vi "RB2 find red 3 dot.vi"(0 "Image In":T1, 1 "error in":errorcluster) -> (2 "Image Out":T1, 3 "Num of\nRed Dots":i32, 4 "Red Dot\nLocation":T2(array[cluster]), 5 "error out":errorcluster)   [LabVIEW 2012]
doc: "This VI find a RED dot on the vehicle in the Mars landscape for Robotics II Spring 2014. It reports the number of Red dots found and their location."
uses:
  <vilib>/vision/Image Controls.llb/IMAQ Image.ctl
  <vilib>/vision/NI_Vision_Development_Module.lvlib
panel:
  out "Mars Result":T1(plugin-control)
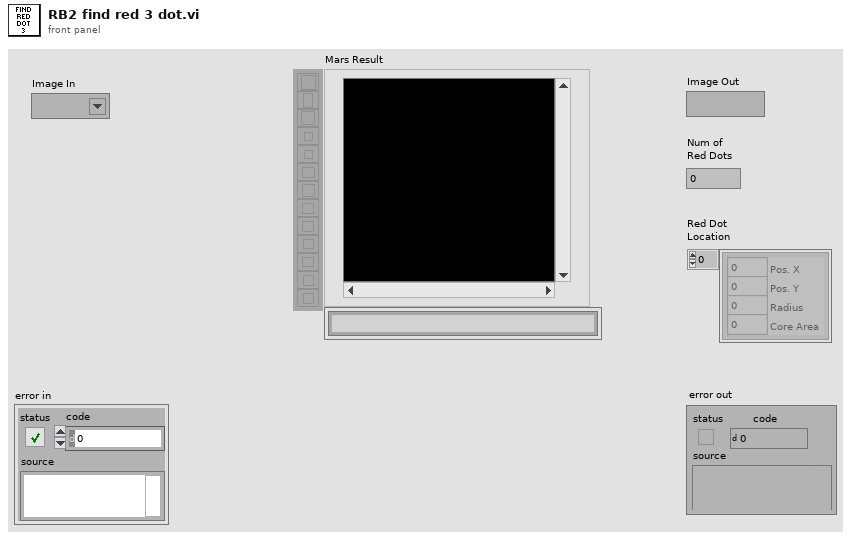
[diagram p1: front panel]
types:
  T1 = typedef "IMAQ Image.ctl" = refnum<image>
  T2 = cluster{"Pos. X":i32, "Pos. Y":i32, "Radius":i32, "Core Area":i32}[]
  T3 = enum32{"AutoM", "Close", "Dilate", "Erode", "Gradient", "Gradient in", "Gradient out", "HitMiss", "Open", "PClose", "POpen", "Thick", "Thin"}
  T4 = typedef "Image Type" = u32
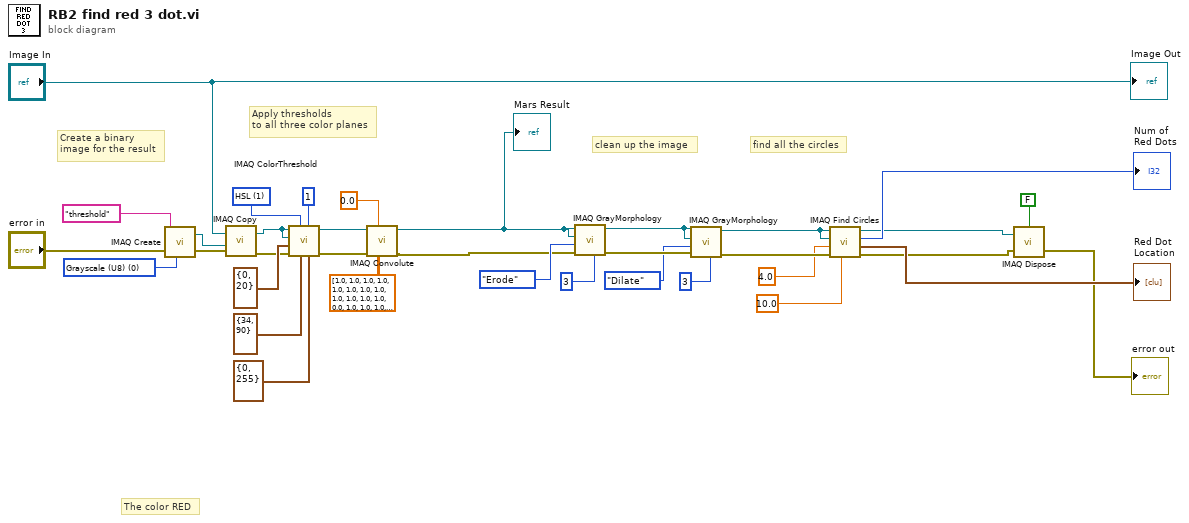
[diagram p0: block diagram]
diagram:
  w12 = u16 1 items=["RGB", "HSL", "HSV", "HSI"] ("Color Mode")
  w32 = T4 0 items=["Grayscale (U8)", "Grayscale (I16)", "Grayscale (SGL)", "Complex (CSG)", "RGB (U32)", "HSL (U32)", "RGB (U64)", "Grayscale (U16)"] ("Image Type")
  # "Create a binary\nimage for the result"
  # "The color RED"
  # "Apply thresholds\nto all three color planes"
  # "find all the circles"
  # "clean up the image"
  n1 = call "IMAQ Create"("Image Name"="threshold", "Image Type"=w32, "error in (no error)"="error in") -> ("New Image"=w34:T1, "error out"=w33:errorcluster)  [unwired: 2 in]
  n2 = call "IMAQ Copy"("error in (no error)"=w33, "Image Dst"=w34, "Image Src"="Image In") -> ("error out"=w3:errorcluster, "Image Dst Out"=w4:T1)  [unwired: 3 in]
  n3 = call "IMAQ ColorThreshold"("Blue or Luma or Val or Inten Range"=cluster{"Lower value":i32, "Upper value":i32} {"Lower value"=0, "Upper value"=255}, "Replace Value"=1, "Green or Sat Range"=cluster{"Lower value":i32, "Upper value":i32} {"Lower value"=34, "Upper value"=90}, "Color Mode"=w12, "error in (no error)"=w3, "Red or Hue Range"=cluster{"Lower value":i32, "Upper value":i32} {"Lower value"=0, "Upper value"=20}, "Image Dst"=w4, "Image Src"=w4) -> ("error out"=w8:errorcluster, "Image Dst Out"=w6:T1)  [unwired: 2 out]
  n4 = call "IMAQ Convolute"("Kernel"=sgl[][] [[1.0, 1.0, 1.0, 1.0, 1.0], [1.0, 1.0, 1.0, 1.0, 1.0], [1.0, 1.0, 0.0, 1.0, 1.0], [1.0, 1.0, 1.0, 1.0, 1.0], [1.0, 1.0, 1.0, 1.0, 1.0]], "Divider (kernel sum)"=sgl 0.0 ("Divider"), "error in (no error)"=w8, "Image Src"=w6) -> ("error out"=w1:errorcluster, "Image Dst Out"=w2:T1)  [unwired: 3 in, 3 out]
  "Mars Result" <- w2
  n5 = call "IMAQ GrayMorphology"("Number of iterations (1)"=3, "error in (no error)"=w1, "Operation"=T3."Erode", "Image Dst"=w2, "Image Src"=w2) -> ("error out"=w29:errorcluster, "Image Dst Out"=w27:T1)  [unwired: 5 in]
  n6 = call "IMAQ GrayMorphology"("Number of iterations (1)"=3, "error in (no error)"=w29, "Operation"=T3."Dilate", "Image Dst"=w27, "Image Src"=w27) -> ("error out"=w24:errorcluster, "Image Dst Out"=w25:T1)  [unwired: 5 in]
  n7 = call "IMAQ Find Circles"("Max Radius"=sgl 10.0, "error in (no error)"=w24, "Min Radius"=sgl 4.0, "Image Dst"=w25, "Image Src"=w25) -> ("error out"=w17:errorcluster, "Circles Data"=→"Red Dot\nLocation":T2, "Nb Circles"=→"Num of\nRed Dots":i32, "Image Dst Out"=w16:T1)  [unwired: 3 in]
  n8 = call "IMAQ Dispose"("All Images? (No)"=FALSE, "Image"=w16, "error in (no error)"=w17) -> ("error out"=→"error out":errorcluster)  [unwired: 3 in]
  "Image Out" <- "Image In"
